vi "A_3.vi"() -> ()   [LabVIEW 2020]
panel:
  in  "Loop delay [ms]":u32=10
  out "LED":bool
  in  "Discrimination level":dbl=2.0 min=-2.0 max=2.0 step=0.01
  in  "Stop":bool
  out "Waveform Chart":cluster{"Dyscrimination level":dbl, dbl}(graph)
  in  "Noise amplitude":dbl
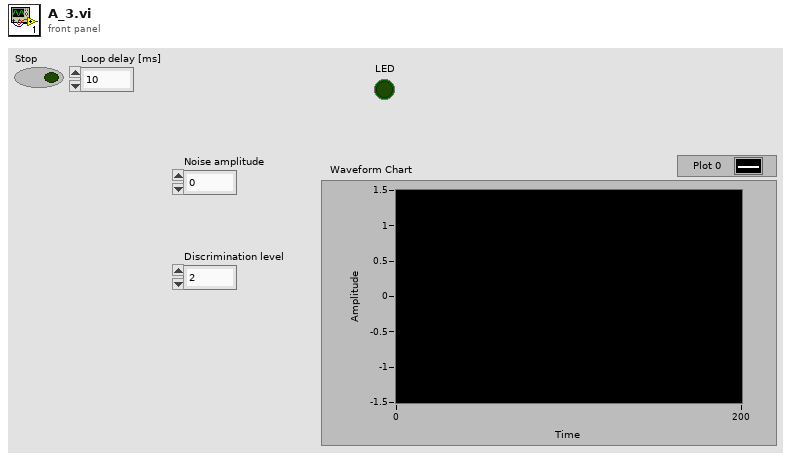
[diagram p1: front panel]
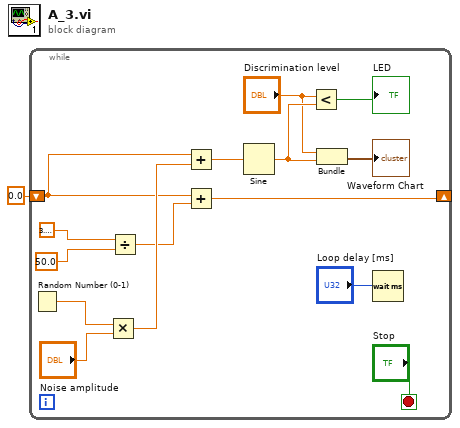
[diagram p0: block diagram]
diagram:
  n1 = while {
    shift-right: [w16] -> _
    shift-left: 0.0 -> [w12]
    stop <- "Stop" stop-if-true
    n2 = Random Number (0-1)() -> (number: 0 to 1=w15:dbl)
    n3 = Multiply(x=w15, y="Noise amplitude") -> (x*y=w13:dbl)
    n4 = Divide(x=3.141592653589793, y=50.0 ("x")) -> (x/y=w9:dbl)
    n5 = Add(x=w12, y=w13) -> (x+y=w11:dbl)
    n6 = Add(x=w12, y=w9) -> (x+y=w16:dbl)
    n7 = Sine(x=w11) -> (sin(x)=w4:dbl)
    n8 = Less?(x="Discrimination level", y=w4) -> (x < y?=→"LED":bool)
    n9 = Bundle("Discrimination level"="Discrimination level", w4) -> (→"Waveform Chart":cluster{"Discrimination level":dbl, dbl})  [unwired: 1 in]
    n10 = Wait (ms)(milliseconds to wait="Loop delay [ms]") -> ()  [unwired: 1 out]
  }
